vi "CH5.vi"() -> ()   [LabVIEW 2021]
panel:
  in  "CH5":cluster{"CH5 Array":dbl[], "CH5 Message":string}
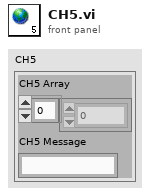
[diagram p1: front panel]
diagram:
